vi "MGI Exit if Runtime.vi"(8 "Error In (Dependency Only)":errorcluster, 11 "VI Reference (Top Level)":refnum<vi>) -> ()   [LabVIEW 2016]
doc: "This VI is designed to be used at the very end of an application that will be run as an executable. It closes the front panel of the executable before exiting LabVIEW, eliminating the annoying flicker as the front panel moves into the non-running state. In source code this VI has no effect.\n\nAuthored by Robert C. Mortensen\nsupport@mooregoodideas.com\nwww.mooregoodideas.com\n\nCopyright (c) 2010, Moore Good Ideas, Inc.\n\nAll rights reserved.\n\nRedistribution and use in source and binary forms, with or without modification, are permitted provided that the following conditions are met:\n\n * Redistributions of source code must retain the above copyright notice, this list of conditions and the following disclaimer.\n * Redistributions in binary form must reproduce the above copyright notice, this list of conditions and the following disclaimer in the documentation and/or other materials provided with the distribution.\n * Neither the name of Moore Good Ideas, Inc. nor the names of its contributors may be used to endorse or promote products derived from this software without specific prior written permission.\n\nTHIS SOFTWARE IS PROVIDED BY THE COPYRIGHT HOLDERS AND CONTRIBUTORS \"AS IS\" AND ANY EXPRESS OR IMPLIED WARRANTIES, INCLUDING, BUT NOT LIMITED TO, THE IMPLIED WARRANTIES OF MERCHANTABILITY AND FITNESS FOR A PARTICULAR PURPOSE ARE DISCLAIMED. IN NO EVENT SHALL THE COPYRIGHT OWNER OR CONTRIBUTORS BE LIABLE FOR ANY DIRECT, INDIRECT, INCIDENTAL, SPECIAL, EXEMPLARY, OR CONSEQUENTIAL DAMAGES (INCLUDING, BUT NOT LIMITED TO, PROCUREMENT OF SUBSTITUTE GOODS OR SERVICES; LOSS OF USE, DATA, OR PROFITS; OR BUSINESS INTERRUPTION) HOWEVER CAUSED AND ON ANY THEORY OF LIABILITY, WHETHER IN CONTRACT, STRICT LIABILITY, OR TORT (INCLUDING NEGLIGENCE OR OTHERWISE) ARISING IN ANY WAY OUT OF THE USE OF THIS SOFTWARE, EVEN IF ADVISED OF THE POSSIBILITY OF SUCH DAMAGE."
uses:
  <userlib>/_MGI/Application Control/MGI VI Reference/MGI Top Level VI Reference.vi
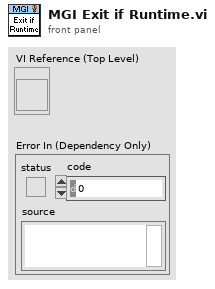
[diagram p1: front panel]
types:
  T1 = enum32{"invalid app kind", "Development System", "Run Time System", "Student Edition", "Embedded LabVIEW", "Evaluation", "Custom"}
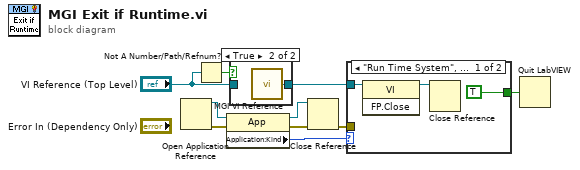
[diagram p0: block diagram]
diagram:
  n1 = Open Application Reference() -> (0:w10:errorcluster, 3:w9:refnum<vi>)  [unwired: 4 in]
  n2 = Not A Number/Path/Refnum?(number/path/refnum="VI Reference (Top Level)") -> (NaN/Path/Refnum?=w4:bool)
  n3 = property class="App"(reference=w9, error in=w10) -> (reference out=w6:refnum<vi>, error out=w7:errorcluster, "Application:Kind"=w8:T1)
  n4 = case shown="True" w4 {
    tunnel: [w11 w12] -> w3
    tunnel: "VI Reference (Top Level)" -> [w11 _]
    frame False {
    }
    frame True {
      n5 = call-poly <userlib>:"MGI VI Reference.vi"() -> ("Top Level VI Reference"=w12:refnum<vi>)  [unwired: 1 in]
    }
  }
  n6 = Close Reference(reference=w6, error in (no error)=w7) -> (error out=w5:errorcluster)
  n7 = case shown="\"Run Time System\", \"Embedded LabVIEW\"" w8 {
    tunnel: w5 -> [_ _]
    tunnel: w3 -> [w14 _]
    tunnel: [TRUE _] -> w1
    frame "Run Time System", "Embedded LabVIEW" {
      n8 = invoke class="VI" method="FP.Close"(reference=w14) -> (reference out=w15:refnum<vi>)  [unwired: 2 in, 2 out]
      n9 = Close Reference(reference=w15) -> ()  [unwired: 1 in, 1 out]
    }
    frame Default {
    }
  }
  n10 = Quit LabVIEW(quit? (T)=w1) -> ()
